vi "Configure Sweep Coupling.vi"(0 "VISA resource name":refnum<visa-resource-name>, 1 "Auto Sweep Time (T: Enable)":bool=TRUE, 2 "Manual Video Bandwidth (3E+6 Hz)":i32=3000000, 3 "Auto Resolution Bandwidth (T: Enable)":bool=TRUE, 5 "Manual Sweep Time (0.3285392 s)":dbl=0.3285392, 7 "Manual VBW/RBW Ratio (1 Hz)":dbl=1.0, 9 "Manual Resolution Bandwidth (3E+6 Hz)":i32=3000000, 11 "error in (no error)":errorcluster, 12 "Auto Video Bandwidth (T: Enable)":bool=TRUE, 13 "Auto VBW/RBW Ratio (T: Enable)":bool=TRUE) -> (4 "VISA resource name out":refnum<visa-resource-name>, 15 "error out":errorcluster)   [LabVIEW 2022 SP3, in "Agilent N934X Series.lvlib"]
doc: "Configures the coupling and sweeping properties of the spectrum analyzer. Resolution bandwidth, video bandwidth, and sweep time can be coupled together by the instrument."
uses:
  <instrlib>/Agilent N934X Series/Agilent N934X Series.lvlib
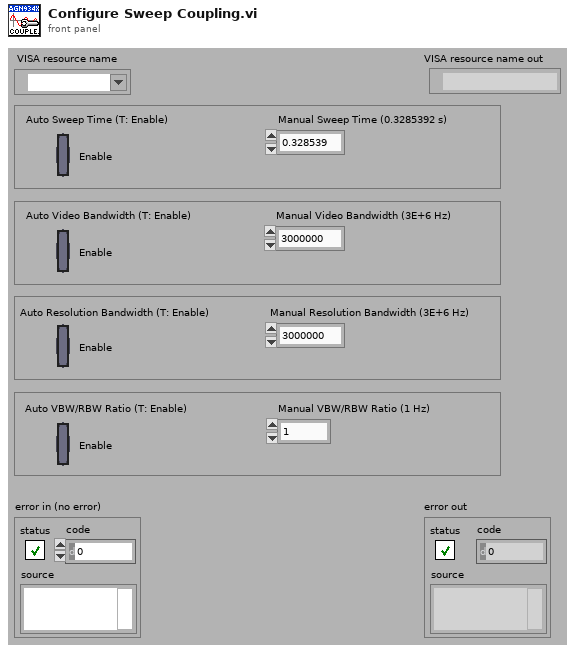
[diagram p1: front panel]
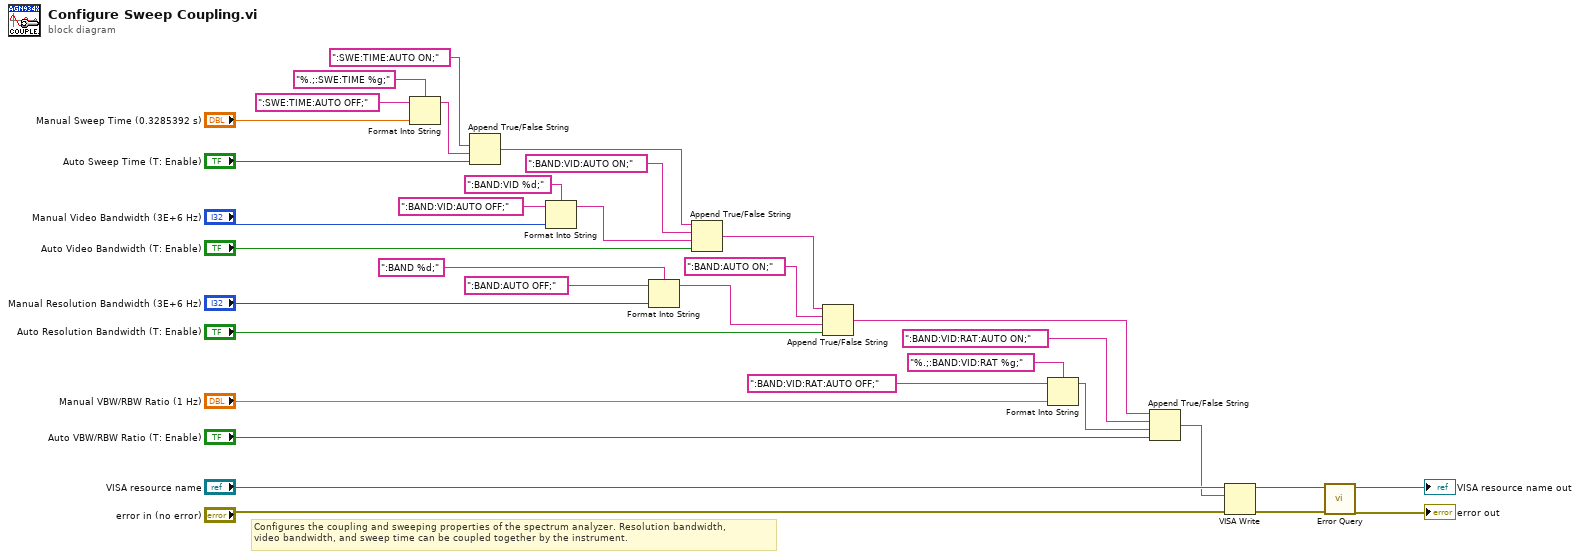
[diagram p0: block diagram]
diagram:
  # "Configures the coupling and sweeping properties of the spectrum analyzer. Resolution bandwidth, \nvideo bandwidth, and sweep time can be coupled together by the instrument."
  n1 = Format Into String(format string="%.;:SWE:TIME %g;", initial string=":SWE:TIME:AUTO OFF;", "Manual Sweep Time (0.3285392 s)") -> (resulting string=w21:string)  [unwired: 1 in, 1 out]
  n2 = Append True/False String(1:"Auto Sweep Time (T: Enable)", 2:w21, 3:":SWE:TIME:AUTO ON;") -> (0:w5:string)  [unwired: 1 in]
  n3 = Format Into String(format string=":BAND:VID %d;", initial string=":BAND:VID:AUTO OFF;", "Manual Video Bandwidth (3E+6 Hz)") -> (resulting string=w18:string)  [unwired: 1 in, 1 out]
  n4 = Format Into String(format string=":BAND %d;", initial string=":BAND:AUTO OFF;", "Manual Resolution Bandwidth (3E+6 Hz)") -> (resulting string=w13:string)  [unwired: 1 in, 1 out]
  n5 = Append True/False String(1:"Auto Video Bandwidth (T: Enable)", 2:w18, 3:":BAND:VID:AUTO ON;", 4:w5) -> (0:w12:string)
  n6 = Append True/False String(1:"Auto Resolution Bandwidth (T: Enable)", 2:w13, 3:":BAND:AUTO ON;", 4:w12) -> (0:w6:string)
  n7 = Format Into String(format string="%.;:BAND:VID:RAT %g;", initial string=":BAND:VID:RAT:AUTO OFF;", "Manual VBW/RBW Ratio (1 Hz)") -> (resulting string=w2:string)  [unwired: 1 in, 1 out]
  n8 = Append True/False String(1:"Auto VBW/RBW Ratio (T: Enable)", 2:w2, 3:":BAND:VID:RAT:AUTO ON;", 4:w6) -> (0:w1:string)
  n9 = VISA Write(VISA resource name="VISA resource name", write buffer=w1, error in (no error)="error in (no error)") -> (VISA resource name out=w28:refnum<visa-resource-name>, error out=w27:errorcluster)  [unwired: 1 out]
  n10 = call <instrlib>:"Error Query.vi"("error in (no error)"=w27, "VISA resource name"=w28) -> ("error out"=→"error out":errorcluster, "VISA resource name out"=→"VISA resource name out":refnum<visa-resource-name>)  [unwired: 6 in, 2 out]
